vi "RSZVB Select More Ratios Generator With Detector.vi"(0 "VISA session":refnum<visa-resource-name>, 1 "Numerator Type (a)":i32(ring) items=["a", "b"], 2 "Denominator Type (a)":i32(ring) items=["a", "b"], 3 "Detector (RMS)":i32(ring) items=["RMS", "Peak", "Average"], 5 "Channel (1)":i32=1, 7 "Trace Name (\"Trc1\")":string="Trc1", 9 "Generator Number (1)":i32=1, 11 "error in (no error)":errorcluster {"code" format="%.0x"}, 12 "Numerator Port Number (1)":i32=1, 13 "Denominator Port Number (1)":i32=1, 14 "Observation Time (0.01)":dbl format="%^.3e") -> (4 "dup VISA session":refnum<visa-resource-name>, 15 "error out":errorcluster {"code" format="%.0x"})   [LabVIEW 2011]
doc: "This VI select arbitrary ratios of wave quantities with detector, e.g. for different detectors and external generator.\n\nAssigns a measurement parameter to an existing trace or creates a trace and assigns a channel number, a name and a measurement parameter to it. The trace is not displayed.\n\nThe notation for ratios and the functionality of the More Ratios dialog is analogous to the definition of S-parameters.\n\nRatio of wave quantities with port numbers and external generator providing the stimulus signal.\n\nRemote-control command(s):\nCALCulate<Ch>:PARameter:SDEFine '<string>', 'B2G1/A1G1SAM' | 'B1G1/A1G1RMS' | 'B2G1/B1G1PEAK' | 'B1G1/B2G1SAM' | ...\nCALCulate<Ch>:PARameter:MEASure '<string>', 'B2G1/A1G1SAM' | 'B1G1/A1G1RMS' | 'B2G1/B1G1PEAK' | 'B1G1/B2G1SAM' | ...\n[SENSe<Ch>:]SWEep:DETector:TIME"
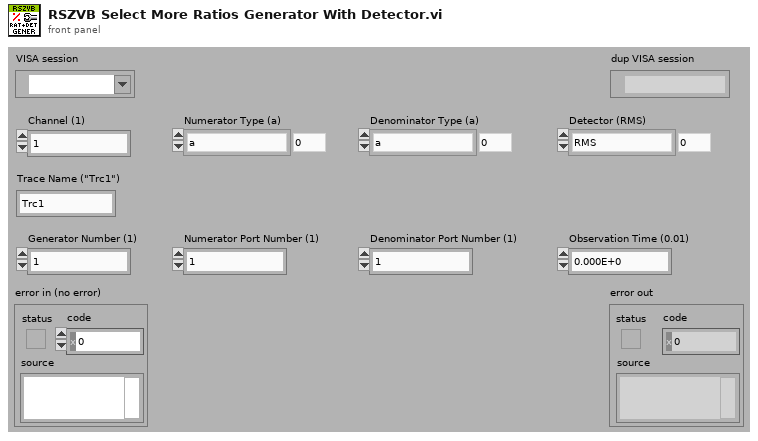
[diagram p1: front panel]
types:
  T1 = cluster{"Error Checking (T: On)":bool, "Installed Options":string[], "Data Valid?":bool, "Ports":i32, "Model":string[], "Option Checking (T: On)":bool}
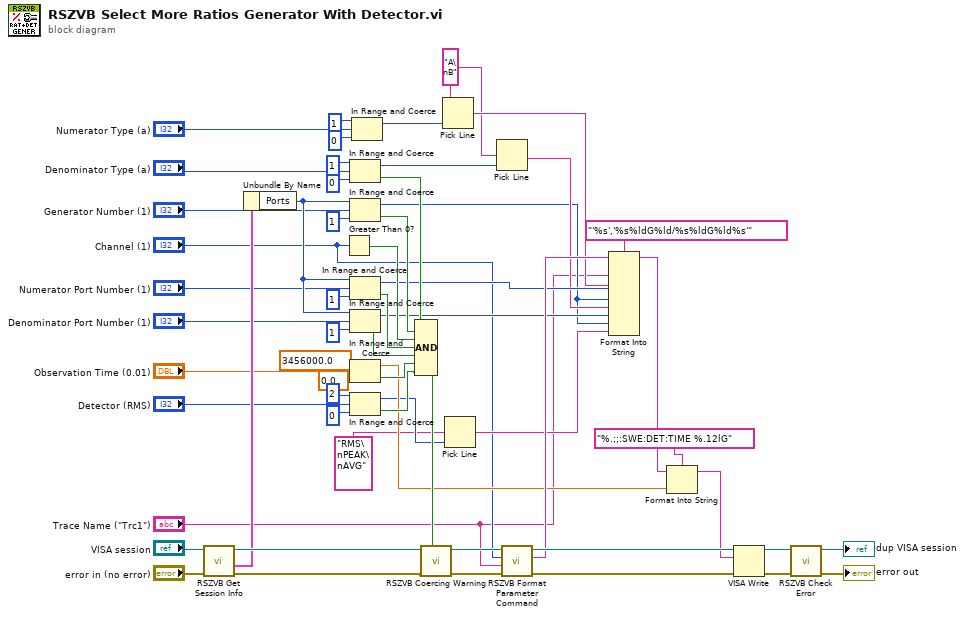
[diagram p0: block diagram]
diagram:
  w34 = "A\nB"
  n1 = call "RSZVB Get Session Info.vi"("error in (no error)"="error in (no error)", "VISA session"="VISA session") -> ("error out"=w18:errorcluster, "Session Info"=w16:T1, "dup VISA session"=w17:refnum<visa-resource-name>)  [unwired: 7 in]
  n2 = Unbundle By Name(w16) -> ("Ports"=w15:i32)
  n3 = Greater Than 0?(x="Channel (1)") -> (x > 0?=w42:bool)
  n4 = In Range and Coerce(upper limit=1, x="Denominator Type (a)", lower limit=0) -> (coerced(x)=w45:i32, In Range?=w44:bool)
  n5 = In Range and Coerce(upper limit=w15, x="Generator Number (1)", lower limit=1) -> (coerced(x)=w31:i32, In Range?=w43:bool)
  n6 = In Range and Coerce(upper limit=w15, x="Numerator Port Number (1)", lower limit=1) -> (coerced(x)=w36:i32, In Range?=w41:bool)
  n7 = In Range and Coerce(upper limit=w15, x="Denominator Port Number (1)", lower limit=1) -> (coerced(x)=w33:i32, In Range?=w40:bool)
  n8 = In Range and Coerce(upper limit=3456000.0, x="Observation Time (0.01)", lower limit=0.0) -> (coerced(x)=w21:dbl, In Range?=w25:bool)
  n9 = In Range and Coerce(upper limit=2, x="Detector (RMS)", lower limit=0) -> (coerced(x)=w20:i32, In Range?=w28:bool)
  n10 = In Range and Coerce(upper limit=1, x="Numerator Type (a)", lower limit=0) -> (coerced(x)=w37:i32)  [unwired: 1 out]
  n11 = Compound Arithmetic op=AND(w44, w43, w42, w41, w40, w25, w28) -> (w55:bool)
  n12 = call "RSZVB Coercing Warning.vi"("In Range?"=w55, "error in (no error)"=w18, "VISA session"=w17) -> ("error out"=w53:errorcluster, "dup VISA session"=w52:refnum<visa-resource-name>)  [unwired: 7 in]
  n13 = Pick Line(multi-line string=w34, line index=w37) -> (output string=w35:string)  [unwired: 1 in]
  n14 = Pick Line(multi-line string="RMS\nPEAK\nAVG", line index=w20) -> (output string=w24:string)  [unwired: 1 in]
  n15 = Pick Line(multi-line string=w34, line index=w45) -> (output string=w32:string)  [unwired: 1 in]
  n16 = call "RSZVB Format Parameter Command.vi"("error in (no error)"=w53, "Trace Name (Trc1)"="Trace Name (\"Trc1\")", "Channel (1)"="Channel (1)", "VISA session"=w52) -> ("error out"=w54:errorcluster, "Buffer"=w49:string, "dup VISA session"=w51:refnum<visa-resource-name>)  [unwired: 5 in]
  n17 = Format Into String(format string="'%s','%s%ldG%ld/%s%ldG%ld%s'", initial string=w49, "Trace Name (\"Trc1\")", w35, w36, w31, w32, w33, w31, w24) -> (resulting string=w23:string)  [unwired: 1 in, 1 out]
  n18 = Format Into String(format string="%.;;:SWE:DET:TIME %.12lG", initial string=w23, w21) -> (resulting string=w22:string)  [unwired: 1 in, 1 out]
  n19 = VISA Write(VISA resource name=w51, write buffer=w22, error in (no error)=w54) -> (VISA resource name out=w56:refnum<visa-resource-name>, error out=w57:errorcluster)  [unwired: 1 out]
  n20 = call "RSZVB Check Error.vi"("error in (no error)"=w57, "VISA session"=w56) -> ("error out"=→"error out":errorcluster, "dup VISA session"=→"dup VISA session":refnum<visa-resource-name>)  [unwired: 8 in]
